vi "Set Cooler ON - OFF.vi"(8 "error in (no error)":errorcluster, 11 "Cooler in":refnum<class "Simulated_Cooler.lvclass">) -> (0 "error out":errorcluster, 3 "Cooler out":refnum<class "Simulated_Cooler.lvclass">)   [LabVIEW 2018, in "Simulated_Cooler.lvclass"]
uses:
  Simulated_Cooler.lvclass
  Simulated_Cooler.lvclass/Simulated_Cooler.ctl
panel:
  out "Cooler ON/OFF":u8
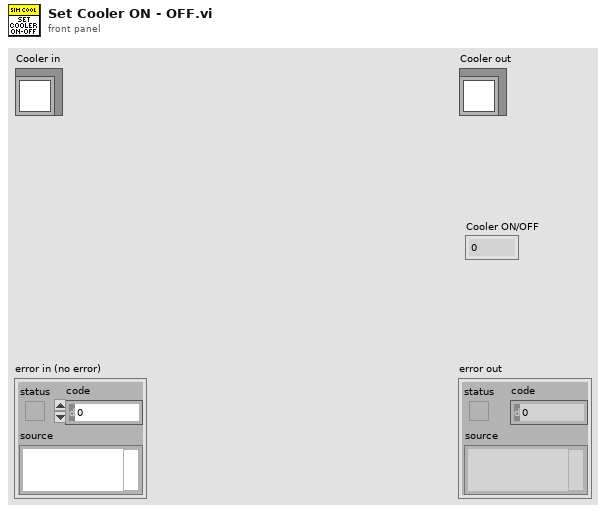
[diagram p1: front panel]
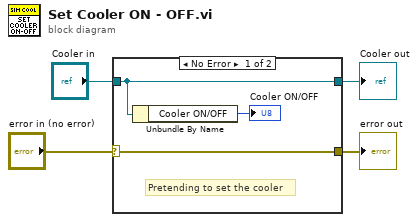
[diagram p0: block diagram]
diagram:
  n1 = case shown="No Error" "error in (no error)" {
    selector: "error in (no error)" -> [w7 w9]
    tunnel: [w7 w9] -> w2
    tunnel: [w6 w8] -> w3
    tunnel: "Cooler in" -> [w6 w8]
    frame No Error {
      # "Pretending to set the cooler"
      n2 = Unbundle By Name(w6) -> ("Cooler ON/OFF"=→"Cooler ON/OFF":u8)
    }
    frame Error {
    }
  }
  "error out" <- w2
  "Cooler out" <- w3
